vi "ProcessDataFlow.vi"(7 "Qbus in":refnum<class "Qbus.lvclass">, 8 "error in (no error)":errorcluster, 10 "Data":T5, 11 "config in":T1) -> (0 "error out":errorcluster, 3 "config out":T1)   [LabVIEW 2017, in "IrTestPanel.lvlib"]
uses:
  <vilib>/addons/InsightCM/Devices/Shared/Ir/IrTestPanel/IrTestPanel.lvlib
  <vilib>/addons/InsightCM/Devices/Shared/Ir/IrTestPanel/controls/config.ctl
  <vilib>/addons/InsightCM/Devices/Shared/Common/TestPanel/controls/Configuration.ctl
  <vilib>/addons/InsightCM/Devices/Shared/Common/TestPanel/controls/State.ctl
  <vilib>/addons/InsightCM/MessageBus/Base/controls/IRoutingSource.ctl
  <vilib>/addons/InsightCM/Devices/Shared/Common/DataFlow/controls/Data.ctl
  <vilib>/addons/InsightCM/Utilities/DataAccessors/controls/wfmSGL_DVR.ctl
  <vilib>/addons/PointValueMap/controls/PointMap.ctl
  <vilib>/addons/InsightCM/Devices/Shared/Common/DataFlow/controls/Type.ctl
  <vilib>/addons/Qbus/Qbus.lvclass
  <vilib>/addons/InsightCM/MessageBus/MessageLibrary/Device/controls/DeviceTestPanelGetDataSetForChannelResponseBody.ctl
  <vilib>/addons/InsightCM/MessageBus/Base/controls/DataSetByteData.ctl
  <vilib>/addons/InsightCM/MessageBus/Base/controls/KeyValuePair.ctl
  <vilib>/addons/InsightCM/Devices/Shared/Common/ServerComm/ServerComm.lvlib
  <vilib>/addons/InsightCM/Devices/Shared/Common/TestPanel/TestPanel.lvlib
  <vilib>/addons/PointValueMap/PointValueMap.lvlib
  <vilib>/addons/InsightCM/Devices/Shared/Common/DataFlow/DataFlow.lvlib
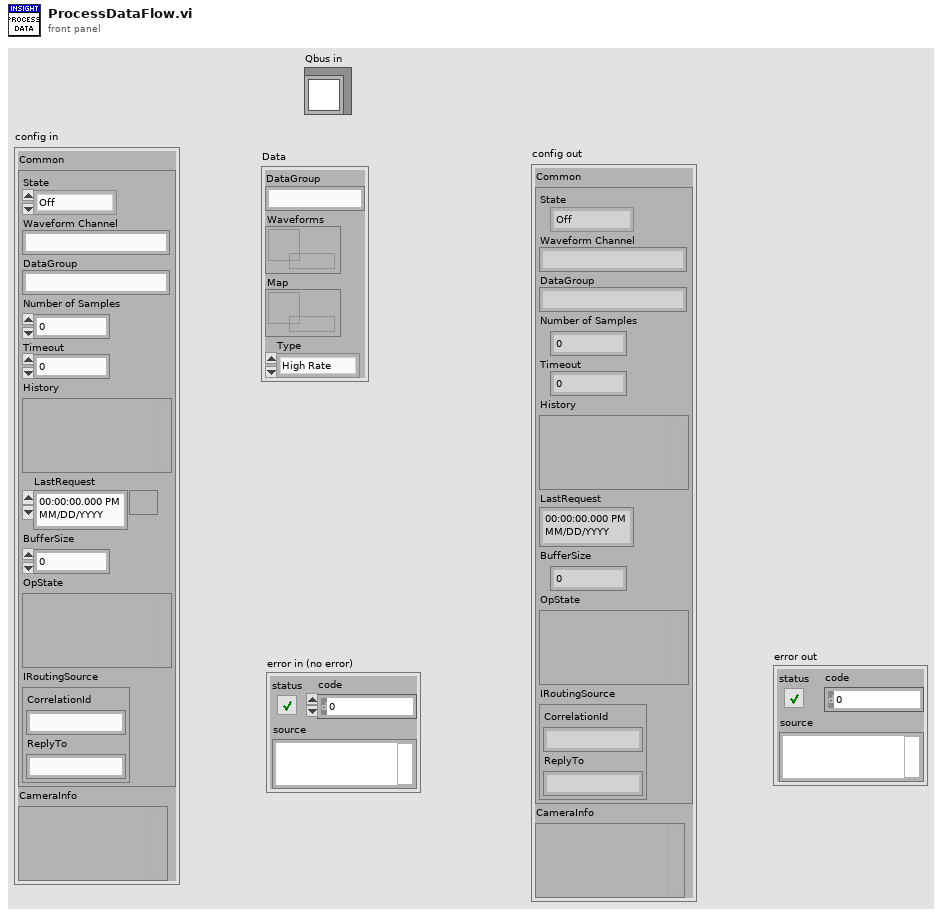
[diagram p1: front panel]
types:
  T1 = typedef "IrTestPanel.lvlib/config.ctl" = cluster{"Common":T2, "CameraInfo":variant}
  T2 = typedef "TestPanel.lvlib/Configuration.ctl" = cluster{"State":T3, "Waveform Channel":string, "DataGroup":string, "Number of Samples":i32, "Timeout":dbl, "History":variant, "LastRequest":timestamp, "BufferSize":i32, "OpState":variant, "IRoutingSource":T4}
  T3 = typedef "TestPanel.lvlib/State.ctl" = enum16{"Off", "On", "PendingValues", "PendingDataSet"}
  T4 = typedef "IRoutingSource.ctl" = cluster{"CorrelationId":string, "ReplyTo":string}
  T5 = typedef "DataFlow.lvlib/Data.ctl" = cluster{"DataGroup":string, "Waveforms":T6, "Map":T7, "Type":T8}
  T6 = typedef "wfmSGL_DVR.ctl" = refnum<data-value>
  T7 = typedef "PointValueMap.lvlib/PointMap.ctl" = refnum<data-value>
  T8 = typedef "DataFlow.lvlib/Type.ctl" = enum16{"High Rate", "Low Rate", "Burst Mode"}
  T9 = typedef "DeviceTestPanelGetDataSetForChannelResponseBody.ctl" = cluster{"DataSet":T10}
  T10 = typedef "DataSetByteData.ctl" = cluster{"Id":string, "DataEventId":string, "AssetNodeId":string, "Type":string, "T0":i64, "Props":T11[], "DataBase64":string}
  T11 = typedef "KeyValuePair.ctl" = cluster{"Key":string, "Value":string}
  T12 = typedef "Message.ctl" = cluster{"Header":T13, "Body":u8[]}
  T13 = typedef "MessageHeader.ctl" = cluster{"MessageName":string, "Timestamp":i64, "CorrelationId":string, "ContentType":string, "RoutingKey":string, "Properties":T11[]}
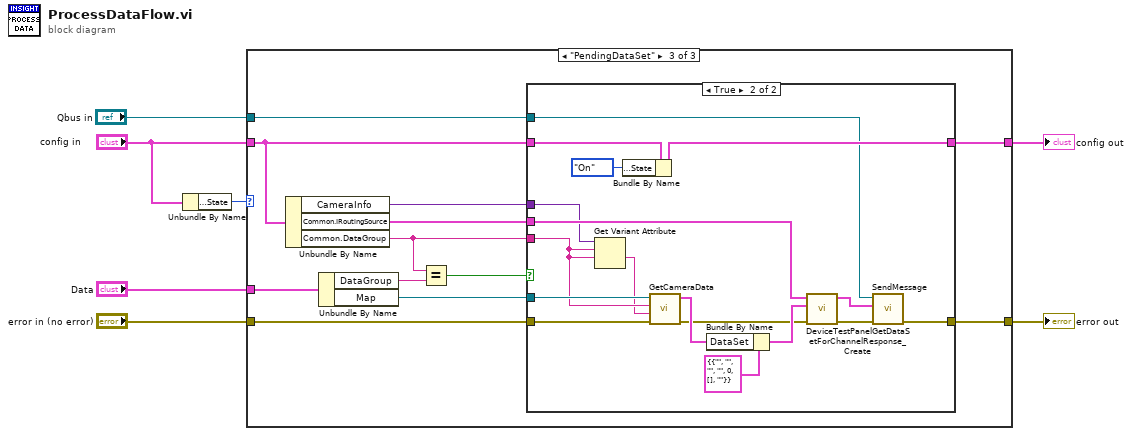
[diagram p0: block diagram]
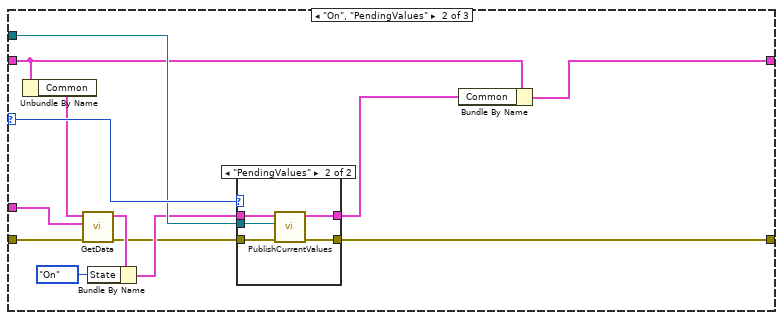
[diagram p3: hidden frame]
diagram:
  n1 = Unbundle By Name("config in") -> ("Common.State"=w7:T3)
  n2 = case shown="\"PendingDataSet\"" w7 {
    selector: w7 -> [_ w22 _]
    tunnel: "error in (no error)" -> [w8 w18 w41]
    tunnel: [w8 w21 w35] -> w2
    tunnel: "config in" -> [w9 w13 w38]
    tunnel: "Data" -> [_ w17 w40]
    tunnel: [w9 w11 w37] -> w3
    tunnel: "Qbus in" -> [_ w20 w36]
    frame "Off" {
    }
    frame "On", "PendingValues" {
      n3 = Unbundle By Name(w13) -> ("Common"=w14:T2)
      n4 = call <vilib>:"GetData.vi"("error in (no error)"=w18, "Data"=w17, "config in"=w14) -> ("error out"=w15:errorcluster, "config out"=w16:T2)  [unwired: 7 in]
      n5 = Bundle By Name(cluster=w16, "State"=State."On" ("Test Panel State")) -> (w19:T2)
      n6 = case shown="\"PendingValues\"" w22 {
        tunnel: w19 -> [w23 w29]
        tunnel: w15 -> [w24 w27]
        tunnel: [w24 w26] -> w21
        tunnel: [w23 w28] -> w12
        tunnel: w20 -> [_ w25]
        frame Default {
        }
        frame "PendingValues" {
          n7 = call <vilib>:"PublishCurrentValues.vi"("error in (no error)"=w27, "Qbus in"=w25, "config in"=w29) -> ("error out"=w26:errorcluster, "config out"=w28:T2)  [unwired: 7 in]
        }
      }
      n8 = Bundle By Name(cluster=w13, "Common"=w12) -> (w11:T1)
    }
    frame "PendingDataSet" {
      n9 = Unbundle By Name(w38) -> ("CameraInfo"=w30:variant, "Common.IRoutingSource"=w31:T4, "Common.DataGroup"=w32:string)
      n10 = Unbundle By Name(w40) -> ("DataGroup"=w34:string, "Map"=w39:T7)
      n11 = Equal?(x=w32, y=w34) -> (x = y?=w33:bool)
      n12 = case shown="True" w33 {
        tunnel: w41 -> [w43 w50]
        tunnel: w39 -> [_ w51]
        tunnel: w38 -> [w42 w60]
        tunnel: [w42 w59] -> w37
        tunnel: w36 -> [_ w58]
        tunnel: [w43 w55] -> w35
        tunnel: w32 -> [_ w45]
        tunnel: w31 -> [_ w47]
        tunnel: w30 -> [_ w46]
        frame False {
        }
        frame True {
          n13 = Get Variant Attribute(Variant=w46, name=w45, default value (empty Variant)=w45) -> (value=w44:string)  [unwired: 1 in, 3 out]
          n14 = Bundle By Name(cluster=w60, "Common.State"=State."On" ("Test Panel State")) -> (w59:T1)
          n15 = call <vilib>:"GetCameraData.vi"("error in (no error)"=w50, "unit"=w44, "Current Camera"=w45, "Map"=w51) -> ("error out"=w48:errorcluster, "DataSet"=w49:T10)  [unwired: 6 in]
          n16 = Bundle By Name(cluster=T9 {"DataSet"={"Id"="", "DataEventId"="", "AssetNodeId"="", "Type"="", "T0"=0, "Props"=[], "DataBase64"=""}} ("DeviceTestPanelGetWaveformChannelResponse"), "DataSet"=w49) -> (w54:T9)
          n17 = call <vilib>:"DeviceTestPanelGetDataSetForChannelResponse_Create.vi"("error in (no error)"=w48, "DeviceTestPanelGetDataSetForChannelResponse"=w54, "IRoutingSource"=w47) -> ("error out"=w56:errorcluster, "Message"=w53:T12)  [unwired: 7 in]
          n18 = call <vilib>:"SendMessage.vi"("error in (no error)"=w56, "message"=w53, "Qbus in"=w58) -> ("error out"=w55:errorcluster)  [unwired: 7 in, 1 out]
        }
      }
    }
  }
  "error out" <- w2
  "config out" <- w3
